vi "Number of Address Map Elements.vi"(2 "DIO":refnum<class "Digital IO.lvclass">) -> (6 "number of elements":u8)   [LabVIEW 2017, in "Digital IO.lvlib" / "Digital IO.lvclass"]
uses:
  Digital IO.lvclass
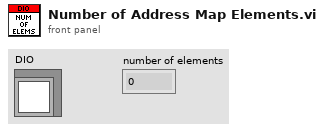
[diagram p1: front panel]
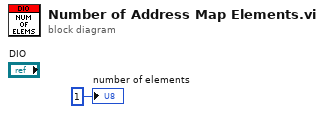
[diagram p0: block diagram]
diagram:
  "number of elements" <- u8 1 ("number of elements")
